vi "UML_Class.vi"(5 "2D Picture in":picture, 6 "Point":refnum<class "Point.lvclass">, 7 "Color":u32(colorbox)=15526085, 8 "error in (no error)":errorcluster, 9 "Methods":string[](array[string])=["Draw ()", "Scale ()", "Move ()"], 10 "Properties":string[](array[string])=["Color : U32"], 11 "Class Name":string="Shape") -> (0 "error out":errorcluster, 2 "2D Picture out":picture, 3 "Collection out":refnum<class "Collection.lvclass">)   [LabVIEW 2021, in "Picture2D.lvlib" / "UMLClass.lvclass"]
uses:
  UMLClass/UMLClass.lvclass
  Collection/Collection.lvclass
  C:/GitHub/Picture2D/src/IDrawable/IDrawable.lvclass
  Point/Point.lvclass
  Text/Text.lvclass
  C:/GitHub/Picture2D/src/Picture2D/Picture2D.lvclass
  2DPictureControl/2DPictureControl.lvclass
  Color/Color.lvclass
  Rectangle/Rectangle.lvclass
  C:/GitHub/Picture2D/src/Shape/Shape.lvclass
  C:/GitHub/Picture2D/src/Polygone/Polygone.lvclass
  PointSpecialized/PointSpecialized.lvclass
  C:/GitHub/Picture2D/src/Point/Point.lvclass
  UMLClass/UMLClass.lvclass/UMLClass.ctl
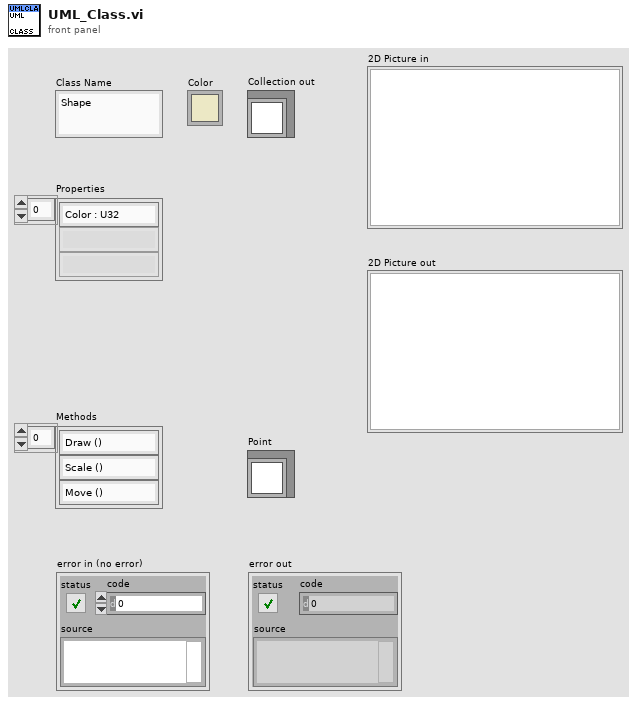
[diagram p1: front panel]
types:
  T1 = cluster{"horizontal":enum16{"left", "center", "right"}, "vertical":enum16{"top", "center", "bottom"}}
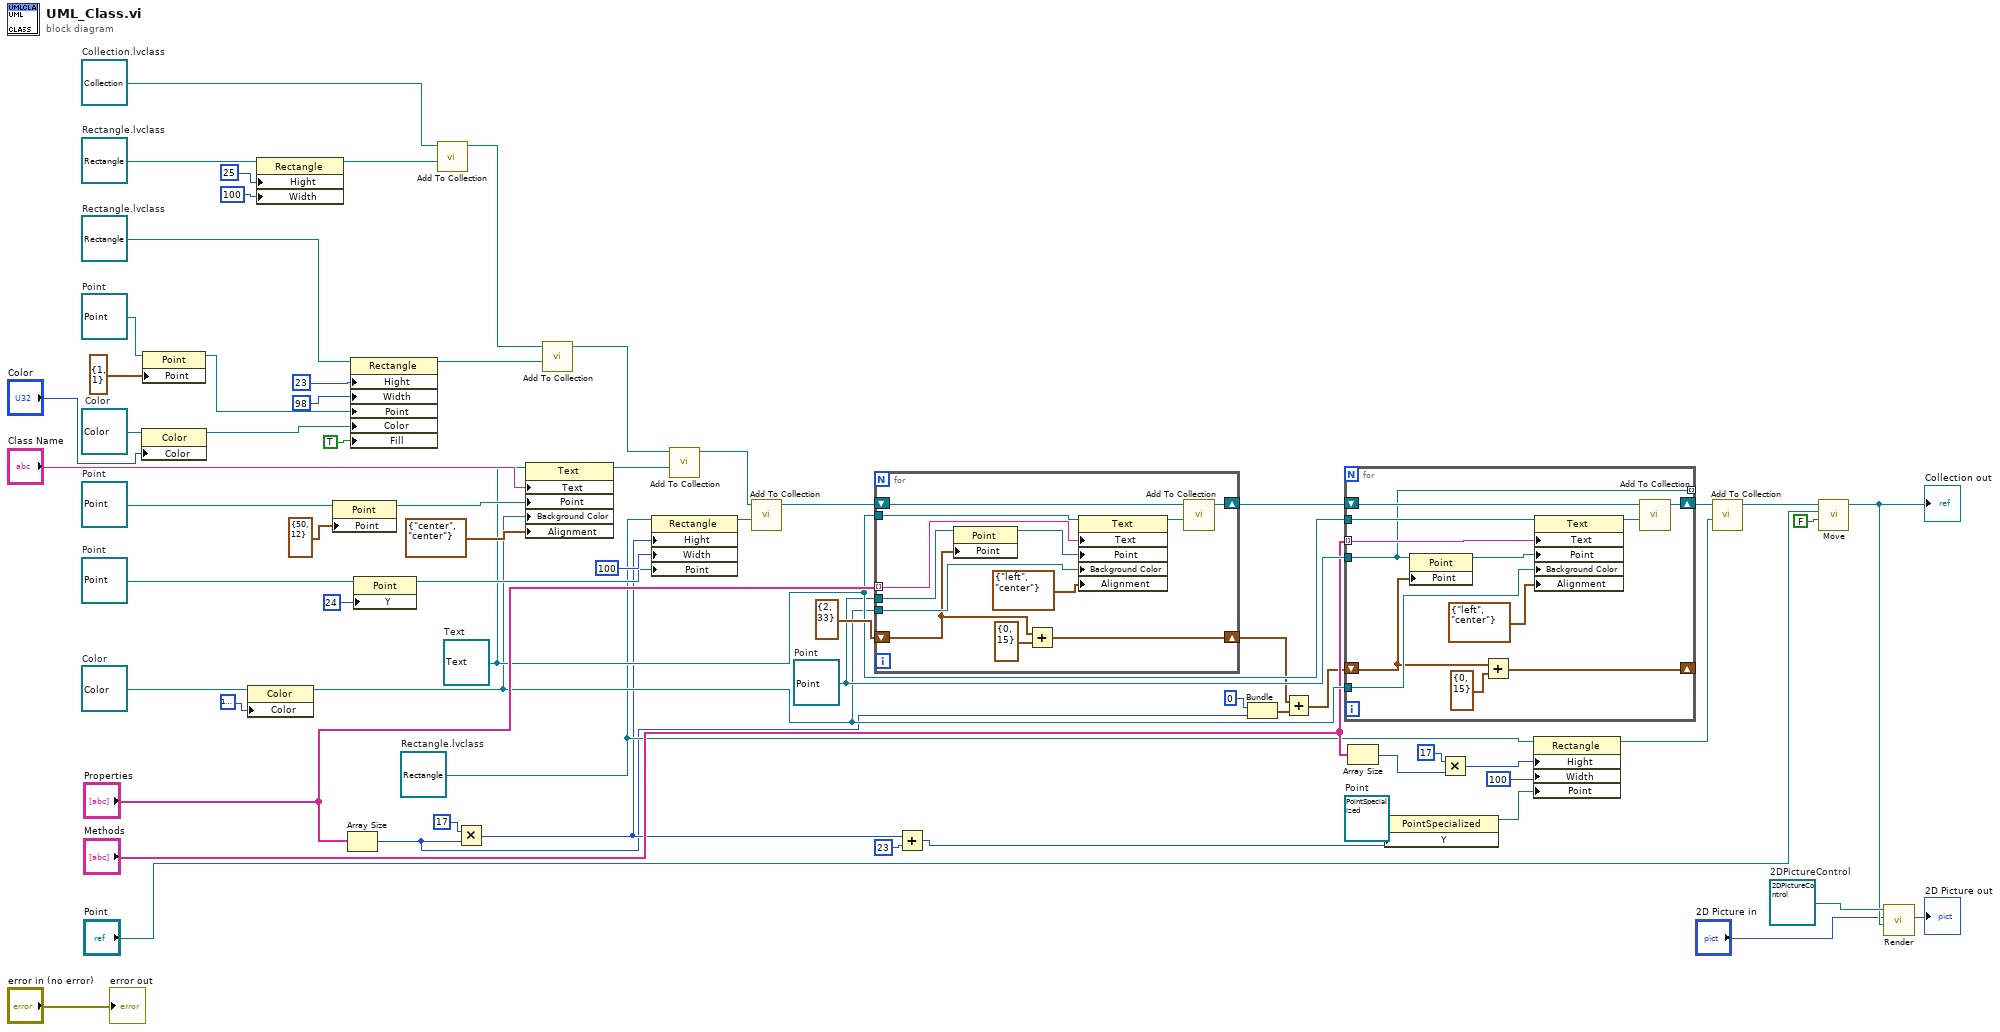
[diagram p0: block diagram]
diagram:
  w5 = refnum<class "Color.lvclass"> refnum  # Color
  w9 = refnum<class "Point.lvclass"> refnum  # Point
  w10 = refnum<class "Rectangle.lvclass"> refnum  # Rectangle.lvclass
  w35 = refnum<class "PointSpecialized.lvclass"> refnum  # Point
  w38 = refnum<class "Point.lvclass"> refnum  # Point
  w48 = refnum<class "Point.lvclass"> refnum  # Point
  w26 = refnum<class "Rectangle.lvclass"> refnum  # Rectangle.lvclass
  w55 = refnum<class "Color.lvclass"> refnum  # Color
  w59 = refnum<class "Point.lvclass"> refnum  # Point
  w66 = refnum<class "2DPictureControl.lvclass"> refnum  # 2DPictureControl
  w39 = refnum<class "Text.lvclass"> refnum  # Text
  w63 = refnum<class "Rectangle.lvclass"> refnum  # Rectangle.lvclass
  w64 = refnum<class "Collection.lvclass"> refnum  # Collection.lvclass
  n1 = property class="Color"(reference=w5, "Color"="Color") -> (reference out=w4:refnum<class "Color.lvclass">)  [unwired: 1 in, 1 out]
  n2 = property class="Point"(reference=w9, "Point"=cluster{"x":i16, "y":i16} {"x"=1, "y"=1} ("Point:All Elements")) -> (reference out=w8:refnum<class "Point.lvclass">)  [unwired: 1 in, 1 out]
  n3 = property class="Color"(reference=w55, "Color"=u32 16777216) -> (reference out=w37:refnum<class "Color.lvclass">)  [unwired: 1 in, 1 out]
  n4 = property class="Rectangle"(reference=w63, "Hight"=i16 25, "Width"=i16 100) -> (reference out=w60:refnum<class "Rectangle.lvclass">)  [unwired: 1 in, 1 out]
  n5 = property class="Point"(reference=w59, "Point"=cluster{"x":i16, "y":i16} {"x"=50, "y"=12} ("Point:All Elements")) -> (reference out=w58:refnum<class "Point.lvclass">)  [unwired: 1 in, 1 out]
  n6 = Array Size(array="Properties") -> (size(s)=w18:i32)
  n7 = property class="Rectangle"(reference=w10, "Hight"=i16 23, "Width"=i16 98, "Point"=w8, "Color"=w4, "Fill"=TRUE) -> (reference out=w6:refnum<class "Rectangle.lvclass">)  [unwired: 1 in, 1 out]
  n8 = property class="Point"(reference=w48, "Y"=i16 24 ("Point:y")) -> (reference out=w47:refnum<class "Point.lvclass">)  [unwired: 1 in, 1 out]
  n9 = call-dynamic "Add To Collection.vi"("IDrawable"=w60, "Collection in"=w64) -> ("Collection out"=w14:refnum<class "Collection.lvclass">)  [unwired: 8 in, 1 out]
  n10 = Multiply(x=i16 17 ("Hight"), y=w18) -> (x*y=w24:i32)
  n11 = property class="Text"(reference=w39, "Text"="Class Name", "Point"=w58, "Background Color"=w37, "Alignment"=T1 {"horizontal"=enum."center", "vertical"=enum."center"}) -> (reference out=w56:refnum<class "Text.lvclass">)  [unwired: 1 in, 1 out]
  n12 = call-dynamic "Add To Collection.vi"("IDrawable"=w6, "Collection in"=w14) -> ("Collection out"=w13:refnum<class "Collection.lvclass">)  [unwired: 8 in, 1 out]
  n13 = property class="Rectangle"(reference=w26, "Hight"=w24, "Width"=i16 100, "Point"=w47) -> (reference out=w49:refnum<class "Rectangle.lvclass">)  [unwired: 1 in, 1 out]
  n14 = call-dynamic "Add To Collection.vi"("IDrawable"=w56, "Collection in"=w13) -> ("Collection out"=w50:refnum<class "Collection.lvclass">)  [unwired: 8 in, 1 out]
  n15 = call-dynamic "Add To Collection.vi"("IDrawable"=w49, "Collection in"=w50) -> ("Collection out"=w40:refnum<class "Collection.lvclass">)  [unwired: 8 in, 1 out]
  n16 = for {
    tunnel: w38 -> [w77]
    tunnel: w37 -> [w75]
    shift-right: [w72] -> w41
    shift-left: w40 -> [w73]
    shift-right: [w69] -> w22
    shift-left: cluster{"x":i16, "y":i16} {"x"=2, "y"=33} ("Point:All Elements") -> [w70]
    tunnel: "Properties" -> [w67] mode=indexing
    tunnel: w39 -> [w78]
    n17 = property class="Point"(reference=w77, "Point"=w70) -> (reference out=w76:refnum<class "Point.lvclass">)  [unwired: 1 in, 1 out]
    n18 = Add(x=w70, y=cluster{"x":i16, "y":i16} {"x"=0, "y"=15} ("Point:All Elements")) -> (x+y=w69:cluster{"x":i16, "y":i16})
    n19 = property class="Text"(reference=w78, "Text"=w67, "Point"=w76, "Background Color"=w75, "Alignment"=T1 {"horizontal"=enum."left", "vertical"=enum."center"}) -> (reference out=w71:refnum<class "Text.lvclass">)  [unwired: 1 in, 1 out]
    n20 = call-dynamic "Add To Collection.vi"("IDrawable"=w71, "Collection in"=w73) -> ("Collection out"=w72:refnum<class "Collection.lvclass">)  [unwired: 8 in, 1 out]
  }
  n21 = Add(x=w24, y=i16 23 ("Point:y")) -> (x+y=w25:i32)
  n22 = Bundle(0, w18) -> (w20:cluster{i32, i32})  [unwired: 1 in]
  n23 = Add(x=w22, y=w20) -> (x+y=w21:cluster{i32, i32})
  n24 = for {
    tunnel: [w79] -> _ mode=indexing
    tunnel: w37 -> [w88]
    shift-right: [w85] -> w29
    shift-left: w41 -> [w86]
    shift-right: [w82] -> _
    shift-left: w21 -> [w83]
    tunnel: "Methods" -> [w80] mode=indexing
    tunnel: w38 -> [w79]
    tunnel: w39 -> [w90]
    n25 = property class="Point"(reference=w79, "Point"=w83) -> (reference out=w89:refnum<class "Point.lvclass">)  [unwired: 1 in, 1 out]
    n26 = Add(x=w83, y=cluster{"x":i16, "y":i16} {"x"=0, "y"=15} ("Point:All Elements")) -> (x+y=w82:cluster{i32, i32})
    n27 = property class="Text"(reference=w90, "Text"=w80, "Point"=w89, "Background Color"=w88, "Alignment"=T1 {"horizontal"=enum."left", "vertical"=enum."center"}) -> (reference out=w84:refnum<class "Text.lvclass">)  [unwired: 1 in, 1 out]
    n28 = call-dynamic "Add To Collection.vi"("IDrawable"=w84, "Collection in"=w86) -> ("Collection out"=w85:refnum<class "Collection.lvclass">)  [unwired: 8 in, 1 out]
  }
  n29 = Array Size(array="Methods") -> (size(s)=w30:i32)
  n30 = property class="PointSpecialized"(reference=w35, "Y"=w25) -> (reference out=w23:refnum<class "PointSpecialized.lvclass">)  [unwired: 1 in, 1 out]
  n31 = Multiply(x=i16 17 ("Hight"), y=w30) -> (x*y=w33:i32)
  n32 = property class="Rectangle"(reference=w26, "Hight"=w33, "Width"=i16 100, "Point"=w23) -> (reference out=w27:refnum<class "Rectangle.lvclass">)  [unwired: 1 in, 1 out]
  n33 = call-dynamic "Add To Collection.vi"("IDrawable"=w27, "Collection in"=w29) -> ("Collection out"=w28:refnum<class "Collection.lvclass">)  [unwired: 8 in, 1 out]
  n34 = call-dynamic "Move.vi"("Absolute (T)"=FALSE, "Point"="Point", "Collection in"=w28) -> ("Collection out"=w17:refnum<class "Collection.lvclass">)  [unwired: 7 in, 1 out]
  "Collection out" <- w17
  n35 = call-dynamic "Render.vi"("IDrawable"=w17, "2D Picture in"="2D Picture in", "2DPictureControl in"=w66) -> ("2D Picture out"=→"2D Picture out":picture)  [unwired: 6 in, 2 out]
  "error out" <- "error in (no error)"
